vi "IMAQ FPGA Camera Link Data to Pixels 2 Tap 8-Bit.vi"(1 "Camera Link Data":cluster{"Port A":u8, "Port B":u8}) -> (0 "Pixels":u8[](array[numeric]))   [LabVIEW 2020]
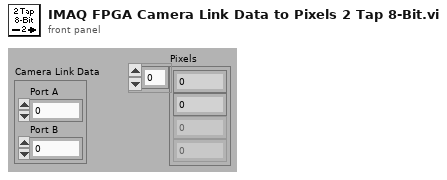
[diagram p1: front panel]
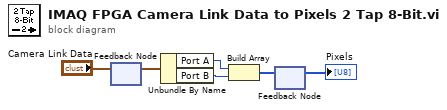
[diagram p0: block diagram]
diagram:
  n1 = feedback #1() -> (w1:cluster{"Port A":u8, "Port B":u8})  [unwired: 1 in]
  n2 = feedback-in #1("Camera Link Data") -> ()
  n3 = Unbundle By Name(w1) -> ("Port A"=w4:u8, "Port B"=w3:u8)
  n4 = Build Array(w4, w3) -> (w6:u8[])
  n5 = feedback-in #2(w6) -> ()
  n6 = feedback #2() -> (→"Pixels":u8[])  [unwired: 1 in]
